vi "Get Channel.vi"(6 "User App":refnum<vi>, 7 "app":refnum<vi>, 10 "Item Path":path, 11 "Element Type":variant) -> (3 "Channel Type":variant)   [LabVIEW 2022 SP3, in "FlexBlocks Support.lvlib"]
uses:
  FlexBlocks Support.lvlib
panel:
  out "error out":errorcluster
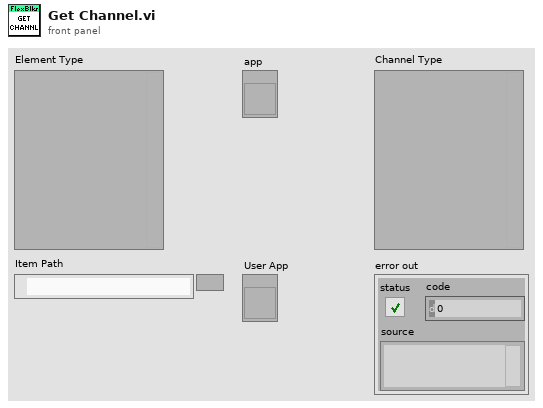
[diagram p1: front panel]
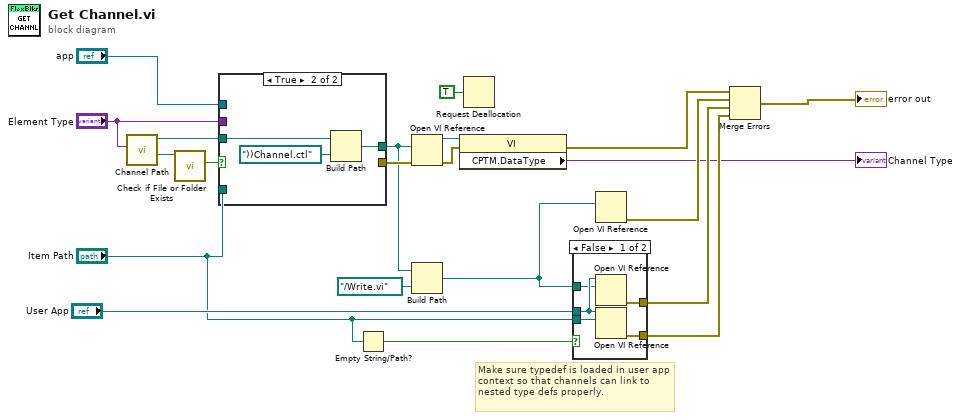
[diagram p0: block diagram]
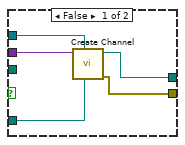
[diagram p3: hidden frame]
diagram:
  # "Make sure typedef is loaded in user app context so that channels can link to nested type defs properly."
  n1 = call "Channel Path.vi"("Variant"="Element Type") -> ("Channel Library Path"=w17:path, "Channel Folder Path"=w16:path)  [unwired: 9 in]
  n2 = call <vilib>:"Check if File or Folder Exists.vi"("path"=w17) -> ("file or folder exists?"=w18:bool)  [unwired: 8 in, 2 out]
  n3 = case shown="True" w18 {
    tunnel: "Element Type" -> [w26 _]
    tunnel: "app" -> [w25 _]
    tunnel: "Item Path" -> [w24 _]
    tunnel: w16 -> [_ w29]
    tunnel: [w23 w27] -> w6
    tunnel: [w22 _] -> w14
    frame False {
      n4 = call "Create Channel.vi"("Item Path"=w24, "app"=w25, "Element Type"=w26) -> ("error IO"=w22:errorcluster, "Channel Control Path"=w23:path)  [unwired: 7 in]
    }
    frame True {
      n5 = Build Path(base path=w29, name or relative path=path "))Channel.ctl") -> (appended path=w27:path)
    }
  }
  n6 = Empty String/Path?(string/path="Item Path") -> (empty?=w10:bool)
  n7 = Open VI Reference(vi path=w6, error in (no error)=w14) -> (vi reference=w19:refnum<vi>, error out=w20:errorcluster)  [unwired: 4 in]
  n8 = Build Path(base path=w6, name or relative path=path "../Write.vi") -> (appended path=w4:path)
  n9 = property class="VI"(reference=w19, error in=w20) -> (error out=w1:errorcluster, "CPTM.DataType"=→"Channel Type":variant)  [unwired: 1 out]
  n10 = Request Deallocation(TRUE ("flag")) -> ()
  n11 = case shown="False" w10 {
    tunnel: "User App" -> [w33 _]
    tunnel: "Item Path" -> [w34 _]
    tunnel: w4 -> [w32 _]
    tunnel: [w31 _] -> w8
    tunnel: [w30 _] -> w7
    frame False {
      n12 = Open VI Reference(application reference (local)=w33, vi path=w32) -> (error out=w31:errorcluster)  [unwired: 4 in, 1 out]
      n13 = Open VI Reference(application reference (local)=w33, vi path=w34) -> (error out=w30:errorcluster)  [unwired: 4 in, 1 out]
    }
    frame True {
    }
  }
  n14 = Open VI Reference(vi path=w4) -> (error out=w3:errorcluster)  [unwired: 5 in, 1 out]
  n15 = Merge Errors(w1, w3, w8, w7) -> (→"error out":errorcluster)
